vi "SRV_Comm_Image.vi"(5 "SRV In":string) -> (0 "error out":errorcluster, 1 "data out":string, 2 "SRV Out":string)   [LabVIEW 2009]
panel:
  # "This LabVIEW item is deprecated.\n\nIt is believed to be unused and will be removed in a future version of SRV."
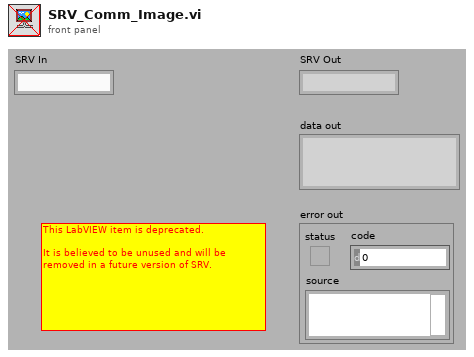
[diagram p1: front panel]
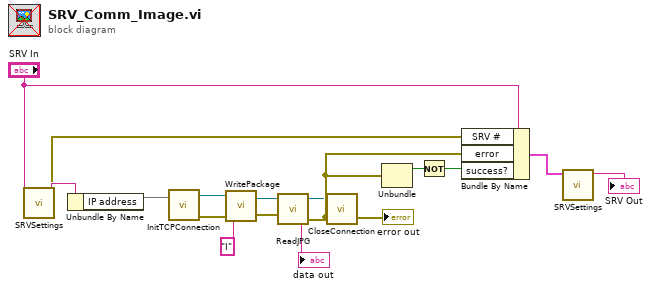
[diagram p0: block diagram]
diagram:
  n1 = call "SRVSettings.vi"("SRV IP Address"="SRV In") -> ("error out"=w15:errorcluster, "SRV IP Address out"=w16:string)  [unwired: 8 in, 1 out]
  n2 = Unbundle By Name(w16) -> ("IP address"=w13)
  n3 = call <userlib>:"InitTCPConnection.vi"("IP address"=w13) -> ("connection ID"=w11:refnum<k5>, "error out"=w12:errorcluster)
  n4 = call <userlib>:"WritePackage.vi"("error in"=w12, "data in"="I", "connection ID in"=w11) -> ("error out"=w6:errorcluster, "connection ID"=w4:refnum<k5>)
  n5 = call <userlib>:"ReadJPG.vi"("error in"=w6, "connection ID in"=w4) -> ("error out"=w5:errorcluster, "data out"=→"data out":string, "connection ID"=w3:refnum<k5>)  [unwired: 1 in]
  "error out" <- w5
  n6 = call <userlib>:"CloseConnection.vi"("error in"=w5, "connection ID"=w3) -> ()  [unwired: 2 in]
  n7 = Unbundle(w5) -> ("status"=w10:bool)  [unwired: 2 out]
  n8 = Not(x=w10) -> (.not. x?=w9:bool)
  n9 = Bundle By Name(cluster="SRV In", "SRV #"=w15, "error"=w5, "success?"=w9) -> (w14:cluster{})
  n10 = call "SRVSettings.vi"("SRV IP Address"=w14) -> ("SRV IP Address out"=→"SRV Out":string)  [unwired: 8 in, 2 out]
